vi "Force Curve_tdms_GetAttributes.vi"(0 "reference in":refnum<class "Force Curve_tdms.lvclass">, 1 "return data? (T)":bool=TRUE, 5 "error in (no error)":errorcluster) -> (14 "reference out":refnum<class "Force Curve_tdms.lvclass">, 15 "attributes ref":T6, 16 "attributes":T1={"MyAttribute"=0.0, "Processed data"=[], "Fcurve Raw Metadata"={"property names"=[], "property values"=[]}, "Fcurve Metadata"={"dt (us)"=0.0, "Dec Factor"=0.0, "Z piezo Sensitivity (nm/V)"=0.0, "K (N/m)"=0.0, "Sp (V)"=0.0, "Contact (ms)"=0.0, "Zpos contact"=0.0, "Vel_app (nm/s)"=0.0, "Vel_ret (nm/s)"=0.0, "deltaV (nm)"=0.0, "Def_V0 (v)"=0.0, "Decimating Factor"=0.0}, "Fcurve index"={"Setpoint index"=2, "Max force index"=2, "Contact point index"=2, "Appoach indices"={"Start"=2, "End"=2}, "Contact indices"={"Start"=2, "End"=2}, "Retract indices"={"Start"=2, "End"=2}}, "Tau Delay (ms)"=0.0, "Contact Spread of dev"=2.0, "Fcurve"={"Approach"={"X"=[], "Y"=[]}, "Contact"={"X"=[], "Y"=[]}, "Retract"={"X"=[], "Y"=[]}}} {"Contact Spread of dev" format="%#_13g"}, 19 "error out":errorcluster)   [LabVIEW 2019, in "Force Curve_tdms.lvclass"]
doc: "Returns a reference and if wanted the actual data values of the attributes. This method is used by the subclasses to access parent attributes."
uses:
  Force Curve_tdms.lvclass
  C:/Program Files (x86)/National Instruments/LabVIEW 2019/vi.lib/addons/_AddQ/G#Object/G#Object.lvclass
  ObjectAttributesRef.ctl
  protected/ObjectAttributes.ctl
  TDMS_DataHandler_class/Fcurve Meta data.ctl
  Fcurve Meta data analysis.ctl
  Fcurve Index .ctl
  Force Curve data.ctl
  Force Curve_tdms.lvclass/Force Curve_tdms.ctl
  <vilib>/addons/_AddQ/G#Object/G#Object.lvclass
  TDMS_DataHandler_class/TDMS_DataHandler.lvclass
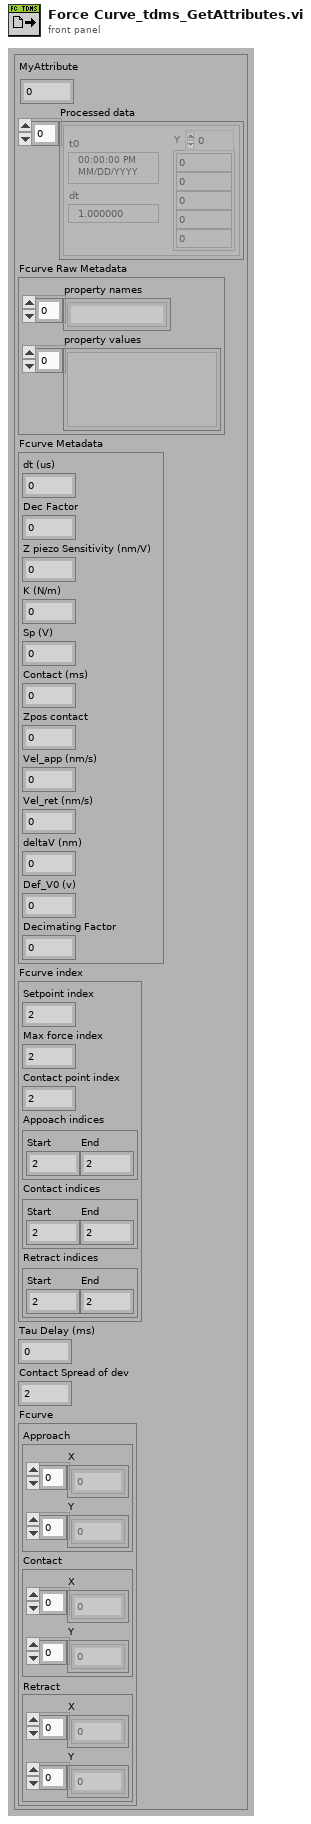
[diagram p1: front panel]
types:
  T1 = typedef "Force Curve_tdms.lvclass/ObjectAttributes.ctl" = cluster{"MyAttribute":dbl, "Processed data":waveform(dbl)[], "Fcurve Raw Metadata":T2, "Fcurve Metadata":T3, "Fcurve index":T4, "Tau Delay (ms)":dbl, "Contact Spread of dev":dbl, "Fcurve":T5}
  T2 = typedef "TDMS_DataHandler.lvclass/Fcurve Meta data.ctl" = cluster{"property names":string[], "property values":variant[]}
  T3 = typedef "Force Curve_tdms.lvclass/Fcurve Meta data analysis.ctl" = cluster{"dt (us)":dbl, "Dec Factor":dbl, "Z piezo Sensitivity (nm/V)":dbl, "K (N/m)":dbl, "Sp (V)":dbl, "Contact (ms)":dbl, "Zpos contact":dbl, "Vel_app (nm/s)":dbl, "Vel_ret (nm/s)":dbl, "deltaV (nm)":dbl, "Def_V0 (v)":dbl, "Decimating Factor":dbl}
  T4 = typedef "Force Curve_tdms.lvclass/Fcurve Index .ctl" = cluster{"Setpoint index":i32, "Max force index":i32, "Contact point index":i32, "Appoach indices":cluster{"Start":i32, "End":i32}, "Contact indices":cluster{"Start":i32, "End":i32}, "Retract indices":cluster{"Start":i32, "End":i32}}
  T5 = typedef "Force Curve_tdms.lvclass/Force Curve data.ctl" = cluster{"Approach":cluster{"X":dbl[], "Y":dbl[]}, "Contact":cluster{"X":dbl[], "Y":dbl[]}, "Retract":cluster{"X":dbl[], "Y":dbl[]}}
  T6 = typedef "Force Curve_tdms.lvclass/ObjectAttributesRef.ctl" = refnum<data-value>
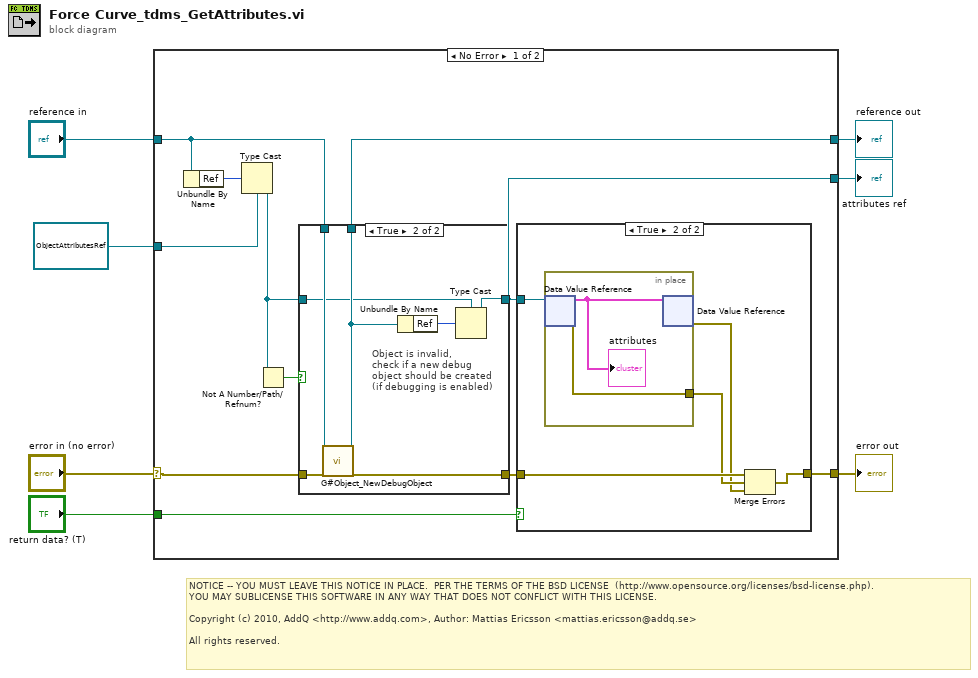
[diagram p0: block diagram]
diagram:
  # "NOTICE -- YOU MUST LEAVE THIS NOTICE IN PLACE.  PER THE TERMS OF THE BSD LICENSE  (http://www.opensource.org/licenses/bsd-license.php).\nYOU MAY SUBLICENSE THIS SOFTWARE IN ANY WAY THAT DOES NOT CONFLICT WITH THIS LICENSE.\n\nCopyright (c) 2010, AddQ <http://www.addq.com>, Author: Mattias Ericsson <mattias.ericsson@addq.se>\n\nAll rights reserved."
  n1 = case shown="No Error" "error in (no error)" {
    selector: "error in (no error)" -> [w14 w39]
    tunnel: [w17 w39] -> w6
    tunnel: [w11 w38] -> w4
    tunnel: "reference in" -> [w12 w38]
    tunnel: [w8 w37] -> w3
    tunnel: "return data? (T)" -> [w18 _]
    tunnel: T6 refnum ("attributes ref") -> [w10 w37]
    frame No Error {
      n2 = Unbundle By Name(w12) -> ("Ref"=w16:u32)
      n3 = Type Cast(type=w10, x=w16) -> (*(type *) &x=w9:T6)
      n4 = Not A Number/Path/Refnum?(number/path/refnum=w9) -> (NaN/Path/Refnum?=w13:bool)
      n5 = case shown="True" w13 {
        tunnel: [w21 w28] -> w15
        tunnel: w14 -> [w21 w27]
        tunnel: w12 -> [w20 w26]
        tunnel: [w20 w24] -> w11
        tunnel: w9 -> [w19 w23]
        tunnel: [w19 w22] -> w8
        frame False {
        }
        frame True {
          # "Object is invalid,\ncheck if a new debug\nobject should be created\n(if debugging is enabled)"
          n6 = call <vilib>:"G#Object_NewDebugObject.vi"("reference in"=w26, "error in (no error)"=w27) -> ("reference out"=w24:refnum<class "Force Curve_tdms.lvclass">, "error out"=w28:errorcluster)  [unwired: 16 in]
          n7 = Unbundle By Name(w24) -> ("Ref"=w25:u32)
          n8 = Type Cast(type=w23, x=w25) -> (*(type *) &x=w22:T6)
        }
      }
      n9 = case shown="True" w18 {
        tunnel: w8 -> [_ w34]
        tunnel: w15 -> [w29 w33]
        tunnel: [w29 w32] -> w17
        frame False {
        }
        frame True {
          n10 = in-place {
            in-place-border: [w36] -> w31
            n11 = in-place-dvr #1(w34) -> (w35:T1, w36:errorcluster)
            "attributes" <- w35
            n12 = in-place-dvr #1(w35) -> (w30:errorcluster)  [unwired: 1 out]
          }
          n13 = Merge Errors(w33, w31, w30) -> (w32:errorcluster)
        }
      }
    }
    frame Error {
    }
  }
  "error out" <- w6
  "reference out" <- w4
  "attributes ref" <- w3
